vi "SetChannels.vi"(8 "error in (no error)":errorcluster, 10 "Channels":T1, 11 "FgenPluginsBase in":refnum<class "FgenPluginsBase.lvclass">) -> (0 "error out":errorcluster, 3 "FgenPluginsBase out":refnum<class "FgenPluginsBase.lvclass">)   [LabVIEW 2014, in "FgenPlugins.lvlib" / "FgenPluginsBase.lvclass"]
uses:
  FgenPluginsBase.lvclass
  TypeDefs/Channels.ctl
  TypeDefs/Channel.ctl
  FgenPluginsBase.lvclass/FgenPluginsBase.ctl
  Accessors/Read Channels.vi
  Accessors/Write Channels.vi
  FgenPlugins.lvlib
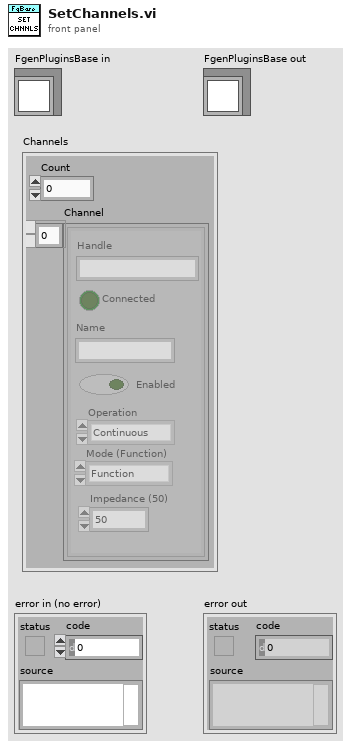
[diagram p1: front panel]
types:
  T1 = typedef "FgenPlugins.lvlib/Channels.ctl" = cluster{"Count":u16, "Channel":T2[]}
  T2 = typedef "FgenPlugins.lvlib/Channel.ctl" = cluster{"Name":string, "Enabled":bool, "Operation":enum16{"Continuous", "Burst"}, "Impedance (50)":dbl, "Handle":string, "Connected":bool, "Mode (Function)":enum16{"Function", "Arbitrary", "Sequence"}}
  T3 = typedef "Channel.ctl" = cluster{"Name":string, "Enabled":bool, "Operation":enum16{"Continuous", "Burst"}, "Impedance (50)":dbl, "Handle":string, "Connected":bool, "Mode (Function)":enum16{"Function", "Arbitrary", "Sequence"}}
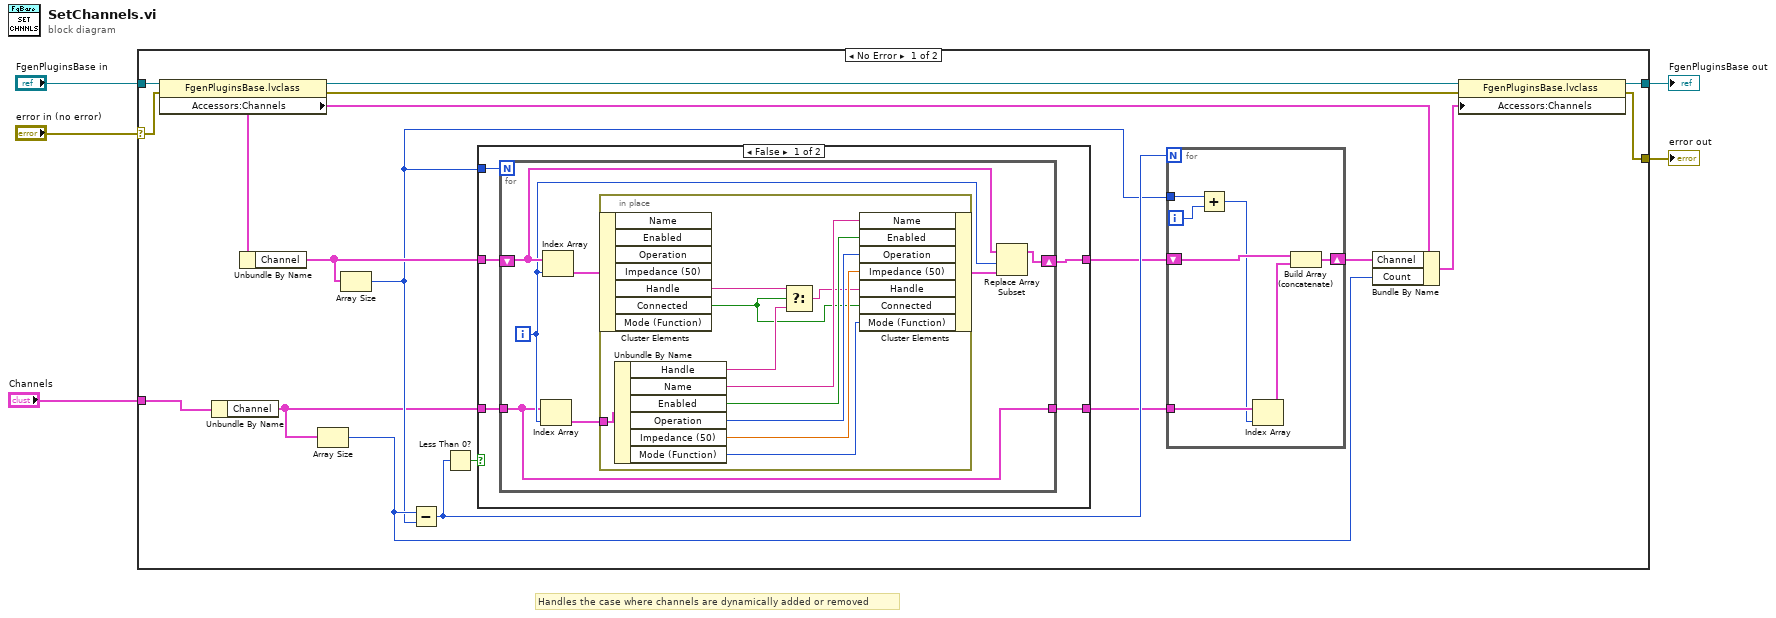
[diagram p0: block diagram]
diagram:
  # "Handles the case where channels are dynamically added or removed"
  n1 = case shown="No Error" "error in (no error)" {
    selector: "error in (no error)" -> [w21 w55]
    tunnel: [w10 w55] -> w4
    tunnel: [w13 w54] -> w2
    tunnel: "FgenPluginsBase in" -> [w23 w54]
    tunnel: "Channels" -> [w20 _]
    frame No Error {
      n2 = property class="FgenPluginsBase.lvclass"(reference=w23, error in=w21) -> (reference out=w22:refnum<class "FgenPluginsBase.lvclass">, error out=w11:errorcluster, "Accessors:Channels"=w15:cluster{"Count":u16, "Channel":T3[]})
      n3 = Unbundle By Name(w20) -> ("Channel"=w6:T2[])
      n4 = Unbundle By Name(w15) -> ("Channel"=w8:T3[])
      n5 = Array Size(array=w6) -> (size(s)=w9:i32)
      n6 = Array Size(array=w8) -> (size(s)=w7:i32)
      n7 = Subtract(x=w9, y=w7) -> (x-y=w18:i32)
      n8 = Less Than 0?(x=w18) -> (x < 0?=w19:bool)
      n9 = case shown="False" w19 {
        tunnel: w8 -> [w35 _]
        tunnel: w6 -> [w34 w53]
        tunnel: w7 -> [w33 _]
        tunnel: [w32 w53] -> w17
        tunnel: [w31 _] -> w16
        frame False {
          n10 = for {
            N: w33 -> [_]
            tunnel: w34 -> [w36]
            shift-right: [w38] -> w32
            shift-left: w35 -> [w41]
            tunnel: [w36] -> w31
            i -> [w39]
            n11 = Index Array(array=w36, index=w39) -> (element=w37:T2)
            n12 = Index Array(array=w41, index=w39) -> (element=w42:T3)
            n13 = in-place {
              in-place-border: w37 -> [w52]
              n14 = in-place-cluster #1(w42) -> ("Handle"=w46:string, "Connected"=w44:bool)  [unwired: 5 out]
              n15 = Unbundle By Name(w52) -> ("Handle"=w45:string, "Name"=w51:string, "Enabled"=w50:bool, "Operation"=w49:enum16{"Continuous", "Burst"}, "Impedance (50)"=w48:dbl, "Mode (Function)"=w47:enum16{"Function", "Arbitrary", "Sequence"})
              n16 = Select(t=w46, s=w44, f=w45) -> (s? t:f=w43:string)
              n17 = in-place-cluster #1("Name"=w51, "Enabled"=w50, "Operation"=w49, "Impedance (50)"=w48, "Handle"=w43, "Connected"=w44, "Mode (Function)"=w47) -> (w40:T3)
            }
            n18 = Replace Array Subset(array=w41, new element=w40, index=w39) -> (w38:T3[])
          }
        }
        frame True {
        }
      }
      n19 = for {
        N: w18 -> [_]
        shift-right: [w26] -> w14
        shift-left: w17 -> [w29]
        tunnel: w16 -> [w28]
        tunnel: w7 -> [w25]
        i -> [w30]
        n20 = Add(x=w25, y=w30) -> (x+y=w27:i32)
        n21 = Index Array(array=w28, index=w27) -> (element=w24:T2)
        n22 = Build Array (concatenate)(w29, w24) -> (w26:T2[])
      }
      n23 = Bundle By Name(cluster=w15, "Channel"=w14, "Count"=w9) -> (w12:cluster{"Count":u16, "Channel":T3[]})
      n24 = property class="FgenPluginsBase.lvclass"(reference=w22, error in=w11, "Accessors:Channels"=w12) -> (reference out=w13:refnum<class "FgenPluginsBase.lvclass">, error out=w10:errorcluster)
    }
    frame Error {
    }
  }
  "error out" <- w4
  "FgenPluginsBase out" <- w2
